vi "sub_upload_parameters.vi"   [LabVIEW 2018]
types:
  T1 = cluster{"VLP16 range setting":refnum<vi>, " VLP16 Mounting Offset":refnum<vi>, "TIM571 Mounting Offset":refnum<vi>, "obstacle limit range":refnum<vi>, "speed cfg":refnum<vi>, "lookahead cfg":refnum<vi>, "Angle cfg":refnum<vi>, "PID limits":refnum<vi>, "PID gains":refnum<vi>, "AGV cfg":refnum<vi>, "waypoint group":refnum<vi>, "PwrPak7 Port":refnum<vi>}
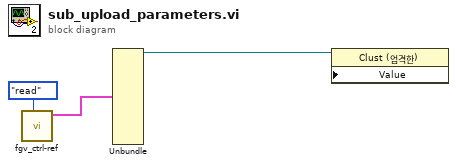
[diagram p0: block diagram]
diagram:
  n1 = call "fgv_ctrl-ref.vi"("cmd"=enum16{"write", "read"}."read") -> ("ref out"=w2:T1)  [unwired: 9 in, 1 out]
  n2 = Unbundle(w2) -> ("VLP16 range setting"=w1:refnum<vi>)  [unwired: 11 out]
  n3 = property class="Clust (엄격한)" props=["Value"](reference=w1) -> ()  [unwired: 2 in, 2 out]
